vi "Shoot.vi"(11 "startShooting":bool) -> (3 "Done":bool)   [LabVIEW 2012]
doc: "Prepares the Shooter for shooting, and shoots once. Accepts Boolean Input: When True, intiates shot; when False, continues in prior state."
panel:
  in  "Use Encoder":bool
  in  "Launch Time":u32=1000
  in  "launchingTime":i32=1000
  in  "launchingSpeed":dbl=4000.0
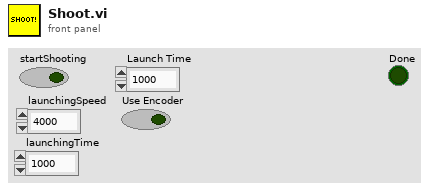
[diagram p1: front panel]
types:
  T1 = enum16{"", "idle", "rotating", "rotating with frisbee"}
  T2 = typedef "WPI_EncoderDevRef.ctl" = cluster{"DevStatus":errorcluster, "EncoderIndex":T3, "CounterIndex":T4, "DistancePerCount":dbl, "Decoding Type":T5}
  T3 = typedef "FPGA_EncoderIdx.ctl" = enum8{"Enc 0", "Enc 1", "Enc 2", "Enc 3", "Invalid"}
  T4 = typedef "FPGA_CounterCtrSystemIndex.ctl" = enum8{"Ctr 0", "Ctr 1", "Ctr 2", "Ctr 3", "Ctr 4", "Ctr 5", "Ctr 6", "Ctr 7", "Invalid"}
  T5 = typedef "WPI_EncoderType.ctl" = enum16{"1x", "2x", "4x"}
  T6 = typedef "WPI_MotorControlDeviceRef.ctl" = cluster{"DeviceStatus":errorcluster, "Type":enum16{"PWM", "CAN"}, "PWM":cluster{"Digital Module":T7, "PWM Channel":T8, "DeadBand":T9}, "CAN":cluster{"Device Number":u8, "Control Mode":T10, "Semaphore":T11, "Max Vout":dbl}, "Invert":bool, "TransformRef":T12, "InvTransformRef":T12}
  T7 = typedef "FPGA_TypedefDigitalModule.ctl" = enum16{"Digital Module 1", "Digital Module 2"}
  T8 = typedef "FPGA_DIOPWMChannel.ctl" = enum8{"PWM 1", "PWM 2", "PWM 3", "PWM 4", "PWM 5", "PWM 6", "PWM 7", "PWM 8", "PWM 9", "PWM 10", "Invalid"}
  T9 = typedef "WPI_PWMDeadband.ctl" = cluster{"Name":string, "maxPositivePwm":i32, "minPositivePwm":i32, "centerPwm":i32, "maxNegativePwm":i32, "minNegativePwm":i32, "angularRange":u16}
  T10 = typedef "WPI_CANJaguar_ControlMode.ctl" = enum8{"Percent VBus", "Current", "Speed", "Position", "Voltage"}
  T11 = typedef "Semaphore RefNum" = refnum<k1>
  T12 = typedef "WPI_PWMTransform_ConPane.ctl" = refnum<vi>
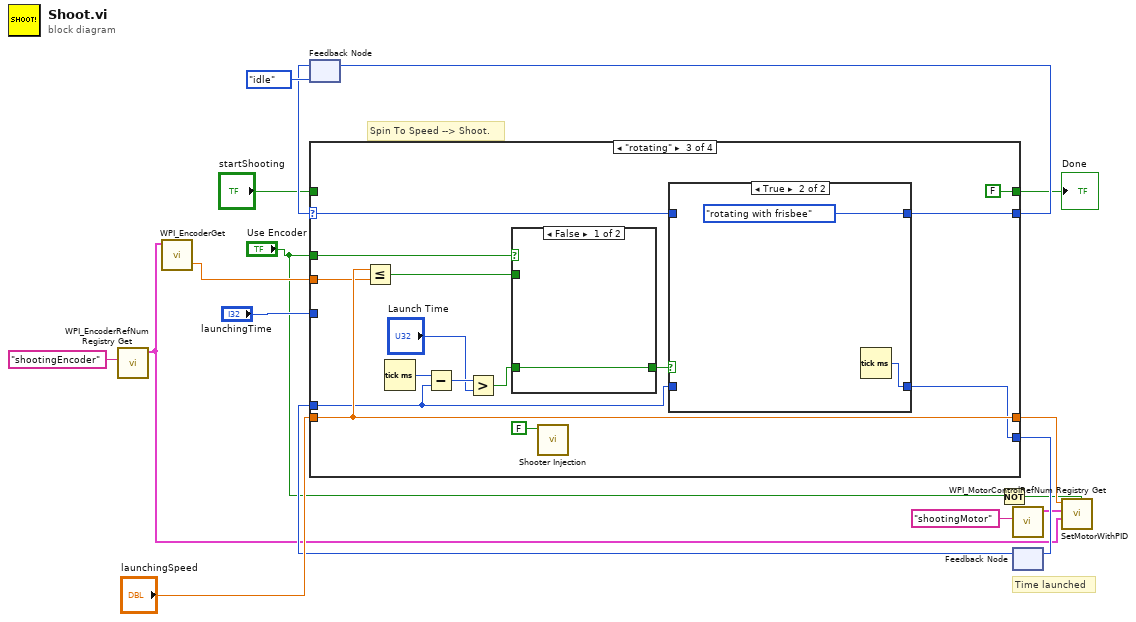
[diagram p0: block diagram]
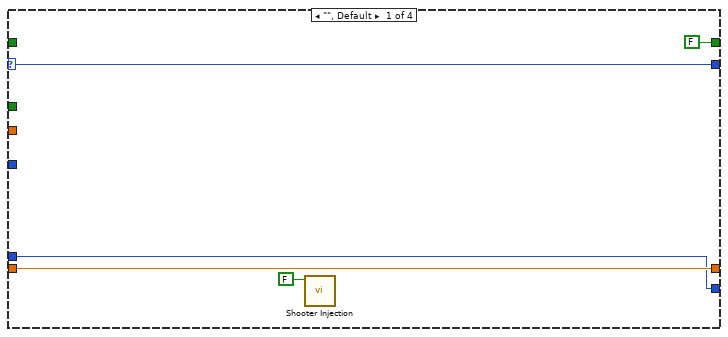
[diagram p2: hidden frame]
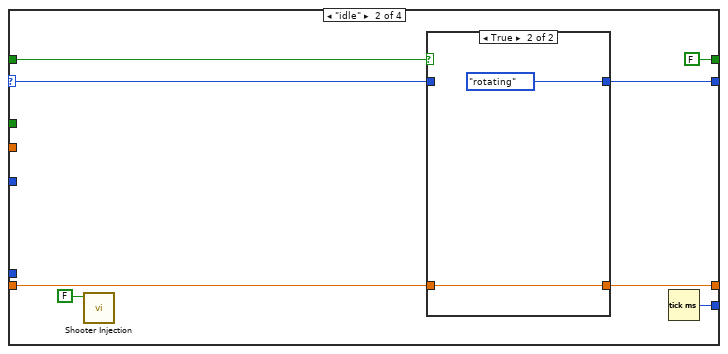
[diagram p3: hidden frame]
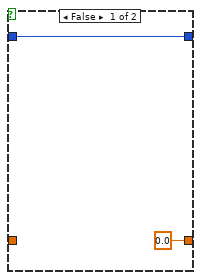
[diagram p4: hidden frame]
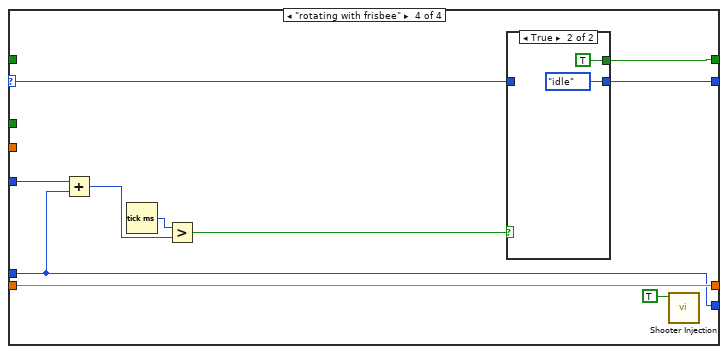
[diagram p7: hidden frame]
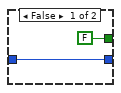
[diagram p8: hidden frame]
diagram:
  # "Time launched"
  # "Spin To Speed --> Shoot."
  n1 = call <vilib>:"WPI_EncoderRefNum Registry Get.vi"("refnum name"="shootingEncoder") -> ("EncoderDevRef"=w4:T2)  [unwired: 9 in, 1 out]
  n2 = call <vilib>:"WPI_EncoderGet.vi"("EncoderDevRef"=w4) -> ("Rate"=w3:dbl)  [unwired: 5 in, 5 out]
  n3 = feedback #1(T1."idle") -> (w16:T1)
  n4 = Not(x="Use Encoder") -> (.not. x?=w2:bool)
  n5 = call <vilib>:"WPI_MotorControlRefNum Registry Get.vi"("refnum name"="shootingMotor") -> ("MotorControlDevRef"=w6:T6)  [unwired: 9 in, 1 out]
  n6 = feedback #2() -> (w10:u32)  [unwired: 1 in]
  n7 = case shown="\"rotating\"" w16 {
    selector: w16 -> [w22 w28 w48 w59]
    tunnel: "startShooting" -> [_ w30 _ _]
    tunnel: [w22 w29 w49 w60] -> w14
    tunnel: "launchingSpeed" -> [w21 w26 w47 w65]
    tunnel: [w21 w27 w47 w65] -> w5
    tunnel: w10 -> [w20 _ w41 w58]
    tunnel: "launchingTime" -> [_ _ _ w64]
    tunnel: [w20 w23 w46 w58] -> w8
    tunnel: [FALSE FALSE FALSE w56] -> w7
    tunnel: w3 -> [_ _ w43 _]
    tunnel: "Use Encoder" -> [_ _ w35 _]
    frame "", Default {
      n8 = call "Shooter Injection.vi"("Inject"=FALSE) -> ()  [unwired: 11 in]
    }
    frame "idle" {
      n9 = call "Shooter Injection.vi"("Inject"=FALSE) -> ()  [unwired: 11 in]
      n10 = case shown="True" w30 {
        tunnel: [w32 T1."rotating"] -> w29
        tunnel: w28 -> [w32 _]
        tunnel: [0.0 w33] -> w27
        tunnel: w26 -> [_ w33]
        frame False {
        }
        frame True {
        }
      }
      n11 = Tick Count (ms)() -> (millisecond timer value=w23:u32)
    }
    frame "rotating" {
      n12 = Less Or Equal?(x=w47, y=w43) -> (x <= y?=w38:bool)
      n13 = Tick Count (ms)() -> (millisecond timer value=w42:u32)
      n14 = Subtract(x=w42, y=w41) -> (x-y=w40:u32)
      n15 = Greater?(x=w40, y="Launch Time") -> (0:w36:bool)
      n16 = case shown="False" w35 {
        tunnel: w38 -> [_ w51]
        tunnel: [w50 w51] -> w37
        tunnel: w36 -> [w50 _]
        frame False {
        }
        frame True {
        }
      }
      n17 = call "Shooter Injection.vi"("Inject"=FALSE) -> ()  [unwired: 11 in]
      n18 = case shown="True" w37 {
        tunnel: [w53 T1."rotating with frisbee"] -> w49
        tunnel: w48 -> [w53 _]
        tunnel: w41 -> [w52 _]
        tunnel: [w52 w54] -> w46
        frame False {
        }
        frame True {
          n19 = Tick Count (ms)() -> (millisecond timer value=w54:u32)
        }
      }
    }
    frame "rotating with frisbee" {
      n20 = Add(x=w64, y=w58) -> (x+y=w62:u32)
      n21 = Tick Count (ms)() -> (millisecond timer value=w63:u32)
      n22 = Greater?(x=w63, y=w62) -> (0:w61:bool)
      n23 = case shown="True" w61 {
        tunnel: [w67 T1."idle"] -> w60
        tunnel: w59 -> [w67 _]
        tunnel: [FALSE TRUE] -> w56
        frame False {
        }
        frame True {
        }
      }
      n24 = call "Shooter Injection.vi"("Inject"=TRUE) -> ()  [unwired: 11 in]
    }
  }
  "Done" <- w7
  n25 = feedback-in #1(w14) -> ()
  n26 = feedback-in #2(w8) -> ()
  n27 = call "SetMotorWithPID.vi"("DisablePID"=w2, "EncoderDevRef"=w4, "MotorControlDeviceRef"=w6, "Speed"=w5) -> ()  [unwired: 7 in, 1 out]
